vi "EncodeFrameHeader.vi"(6 "HeaderLen":i32=2, 8 "ErrorIn":errorcluster, 10 "Header":string="FS", 11 "FrameIn":string) -> (0 "ErrorOut":errorcluster, 3 "FrameOut":string)   [LabVIEW 2016]
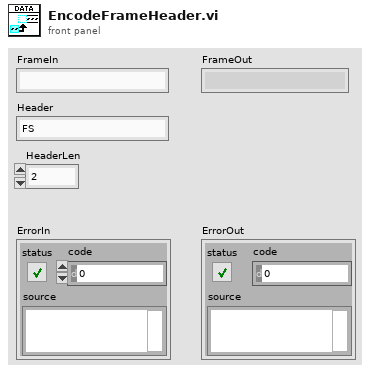
[diagram p1: front panel]
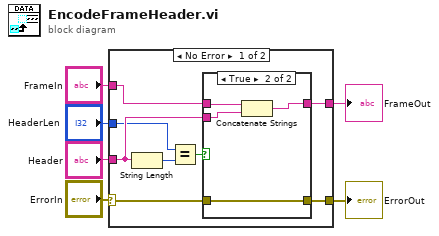
[diagram p0: block diagram]
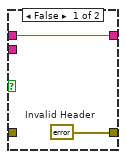
[diagram p2: hidden frame]
diagram:
  n1 = case shown="No Error" "ErrorIn" {
    selector: "ErrorIn" -> [w12 w22]
    tunnel: [w14 w22] -> w6
    tunnel: "Header" -> [w8 _]
    tunnel: "HeaderLen" -> [w7 _]
    tunnel: "FrameIn" -> [w10 w21]
    tunnel: [w9 w21] -> w1
    frame No Error {
      n2 = String Length(string=w8) -> (length=w11:i32)
      n3 = Equal?(x=w7, y=w11) -> (x = y?=w13:bool)
      n4 = case shown="True" w13 {
        tunnel: w12 -> [_ w20]
        tunnel: [w16 w20] -> w14
        tunnel: w10 -> [w15 w19]
        tunnel: [w15 w17] -> w9
        tunnel: w8 -> [_ w18]
        frame False {
          w16 = errorcluster {"status"=TRUE, "code"=2, "source"="Invalid Header"}  # Invalid Header
        }
        frame True {
          n5 = Concatenate Strings(w19, w18) -> (w17:string)
        }
      }
    }
    frame Error {
    }
  }
  "ErrorOut" <- w6
  "FrameOut" <- w1
